vi "CleanUp.vi"(0 "object in":refnum<class "TowerLight.lvclass">, 5 "error in (no error)":errorcluster) -> (14 "object out":refnum<class "TowerLight.lvclass">, 19 "error out":errorcluster)   [LabVIEW 2014, in "TowerLight.lvclass"]
uses:
  TowerLight.lvclass
  TowerLight.lvclass/TowerLight.ctl
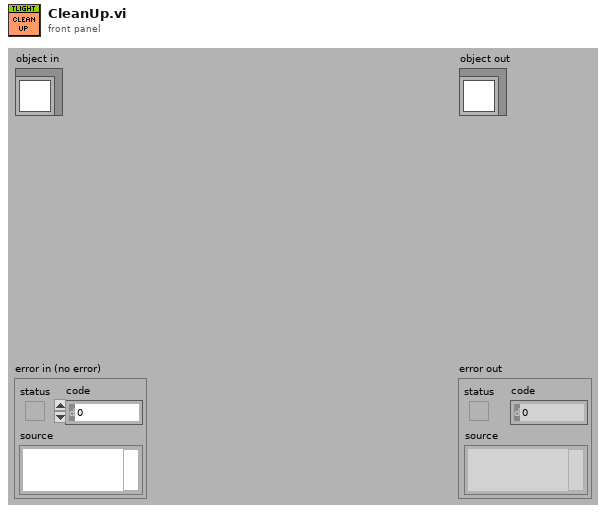
[diagram p1: front panel]
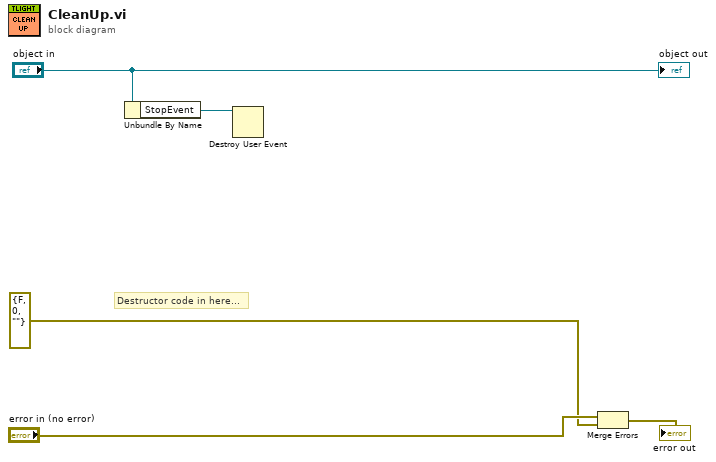
[diagram p0: block diagram]
diagram:
  # "Destructor code in here..."
  n1 = Unbundle By Name("object in") -> ("StopEvent"=w1:refnum<user-event>)
  n2 = Destroy User Event(user event=w1) -> ()  [unwired: 1 in, 1 out]
  n3 = Merge Errors("error in (no error)", errorcluster {"status"=FALSE, "code"=0, "source"=""} ("error in (no error)")) -> (→"error out":errorcluster)
  "object out" <- "object in"
